vi "adsr_decay.vi"(6 "Decay":dbl(knob) scale=0.05..0.001, 8 "error in (no error)":errorcluster, 10 "Number of samples":i32, 11 "Current Amplitude":dbl) -> (0 "error out":errorcluster, 2 "Current amplitude":dbl, 3 "Ramp Pattern":dbl[](array[numeric]))   [LabVIEW 2024]
uses:
  <vilib>/Analysis/1siggen.llb/Ramp Pattern by Samples.vi
  <vilib>/Analysis/NI_AALBase.lvlib
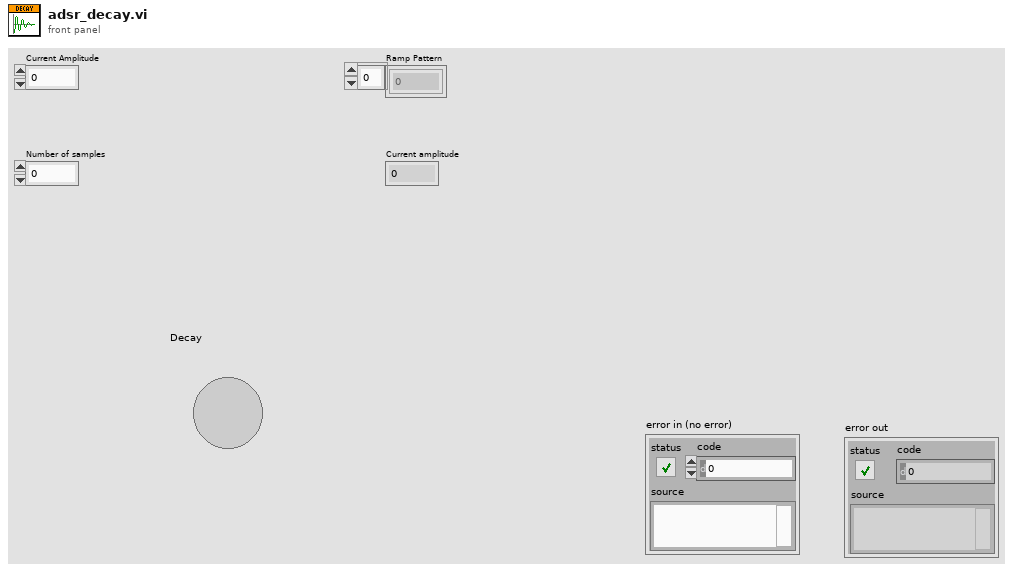
[diagram p1: front panel]
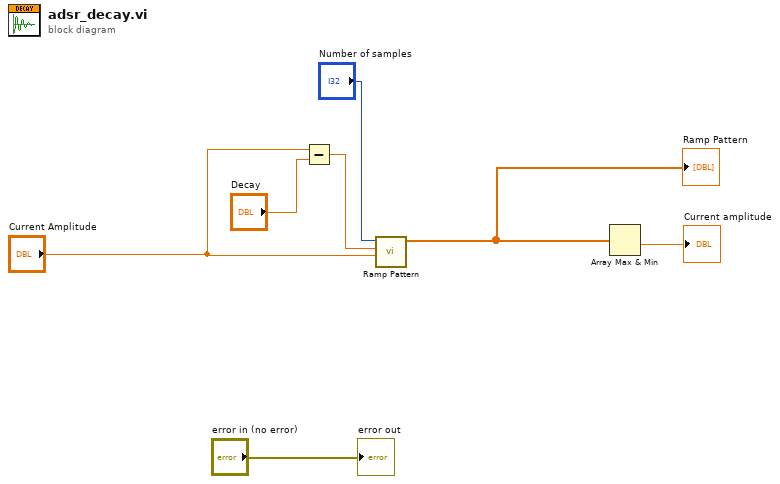
[diagram p0: block diagram]
diagram:
  n1 = Subtract(x="Current Amplitude", y="Decay") -> (x-y=w3:dbl)
  n2 = call-poly <vilib>:"Ramp Pattern.vi"("start"="Current Amplitude", "end"=w3, "samples"="Number of samples") -> ("Ramp Pattern"=w6:dbl[])  [unwired: 7 in, 1 out]
  "Ramp Pattern" <- w6
  n3 = Array Max & Min(array=w6) -> (min value=→"Current amplitude":dbl)  [unwired: 3 out]
  "error out" <- "error in (no error)"
